vi "TruncateConcentrationAccordingToMultipleChargeDistribution.vi"(2 "Sizes":dbl[](array[numeric]), 3 "Concentration":dbl[](array[numeric])) -> (0 "Truncated Sizes":dbl[](array[numeric]), 1 "Truncated Concentration":dbl[](array[numeric]))   [LabVIEW 2011]
uses:
  <vilib>/Analysis/NI_AAL_SigProc.lvlib
panel:
  out "Location with new algorithm":i32
  out "Peak":dbl[](array[numeric])
  out "Location":dbl
  out "Extinction Graph 2":cluster{"Sizes":dbl[], "Amplitudes":dbl[]}[](graph)
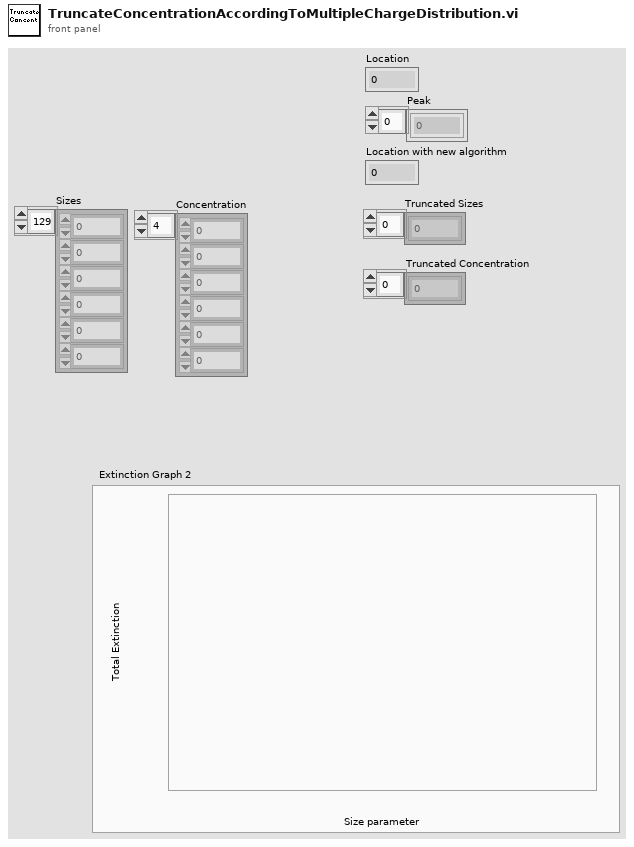
[diagram p1: front panel]
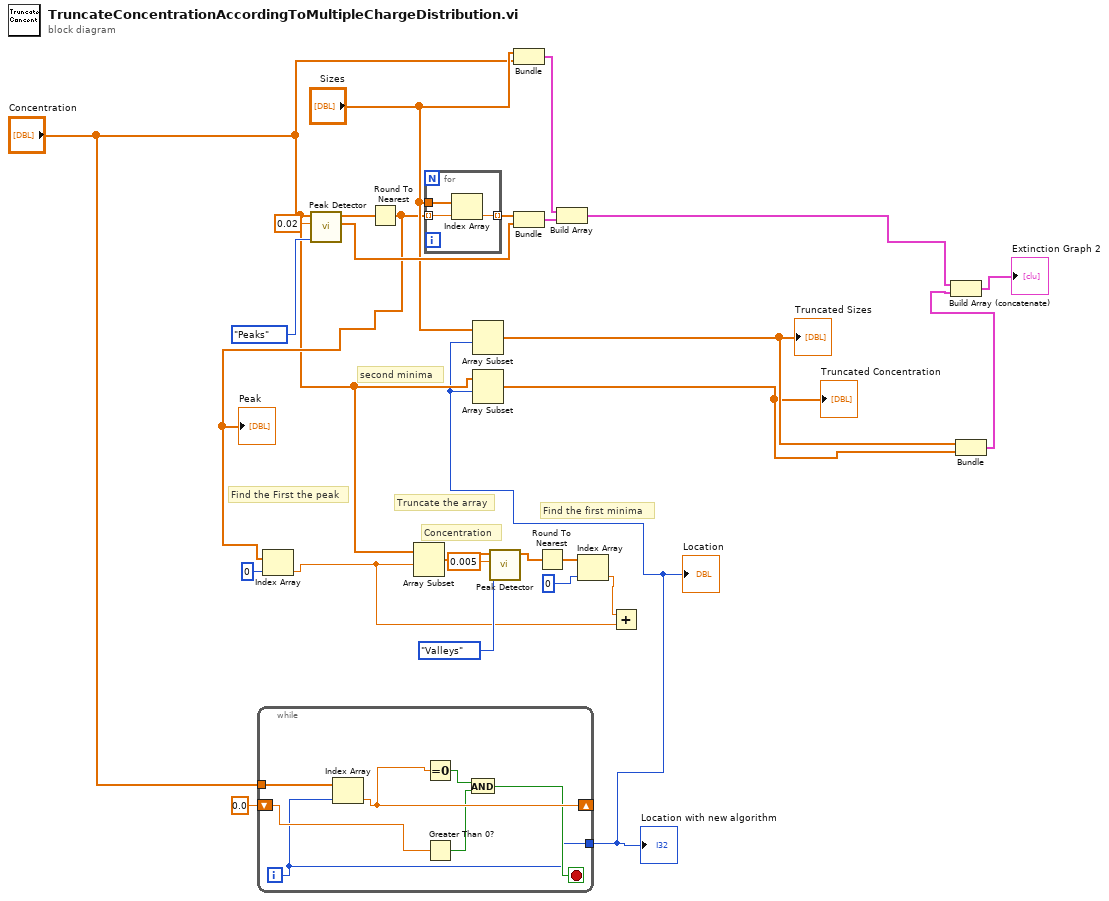
[diagram p0: block diagram]
diagram:
  # "Concentration"
  # "Find the first minima"
  # "Truncate the array"
  # "Find the First the peak"
  # "second minima"
  n1 = while {
    shift-right: [w31] -> _
    shift-left: 0.0 -> [w32]
    tunnel: "Concentration" -> [w33]
    tunnel: [w27] -> w1
    i -> [w27]
    stop <- w28 stop-if-true
    n2 = Index Array(array=w33, index=w27) -> (element=w31:dbl)
    n3 = Equal To 0?(x=w31) -> (x = 0?=w30:bool)
    n4 = Greater Than 0?(x=w32) -> (x > 0?=w29:bool)
    n5 = And(x=w30, y=w29) -> (x .and. y?=w28:bool)
  }
  "Location" <- w1
  "Location with new algorithm" <- w1
  n6 = call <vilib>:"Peak Detector.vi"("peaks/valleys"=enum32{"Peaks", "Valleys"}."Peaks", "threshold"=0.02, "X"="Concentration") -> ("Amplitudes"=w21:dbl[], "Locations"=w23:dbl[])  [unwired: 4 in, 3 out]
  n7 = Round To Nearest(number=w23) -> (nearest integer value=w4:dbl[])
  "Peak" <- w4
  n8 = Index Array(array=w4, index=0) -> (element=w7:dbl)
  n9 = Array Subset(array="Concentration", index=w7) -> (w13:dbl[])  [unwired: 1 in]
  n10 = for {
    tunnel: "Sizes" -> [w36]
    tunnel: w4 -> [w35] mode=indexing
    tunnel: [w34] -> w22 mode=indexing
    n11 = Index Array(array=w36, index=w35) -> (element=w34:dbl)
  }
  n12 = Array Subset(array="Sizes", index=w1) -> (w26:dbl[])  [unwired: 1 in]
  "Truncated Sizes" <- w26
  n13 = Array Subset(array="Concentration", index=w1) -> (w17:dbl[])  [unwired: 1 in]
  "Truncated Concentration" <- w17
  n14 = call <vilib>:"Peak Detector.vi"("peaks/valleys"=enum32{"Peaks", "Valleys"}."Valleys", "threshold"=0.005, "X"=w13) -> ("Locations"=w10:dbl[])  [unwired: 4 in, 4 out]
  n15 = Bundle("Sizes"="Sizes", "Concentration"="Concentration") -> (w20:cluster{"Sizes":dbl[], "Concentration":dbl[]})  [unwired: 1 in]
  n16 = Bundle(w22, "Amplitudes"=w21) -> (w19:cluster{dbl[], "Amplitudes":dbl[]})  [unwired: 1 in]
  n17 = Round To Nearest(number=w10) -> (nearest integer value=w9:dbl[])
  n18 = Build Array(w20, w19) -> (w25:cluster{"Sizes":dbl[], "Amplitudes":dbl[]}[])
  n19 = Index Array(array=w9, index=0) -> (element=w8:dbl)
  n20 = Add(x=w8, y=w7) -> ()  [unwired: 1 out]
  n21 = Bundle(w26, w17) -> (w16:cluster{dbl[], dbl[]})  [unwired: 1 in]
  n22 = Build Array (concatenate)(w25, w16) -> (→"Extinction Graph 2":cluster{"Sizes":dbl[], "Amplitudes":dbl[]}[])
